vi "Disconnect.vi"(8 "Error In":errorcluster, 11 "Agent In":refnum<class "Agent.lvclass">) -> (0 "Error Out":errorcluster, 3 "Agent Out":refnum<class "Agent.lvclass">)   [LabVIEW 2018, in "Toolkit.lvlib" / "Agent.lvclass"]
doc: "Disconnects and closes the connection to the SSH agent application. This should be called before the Agent object is destroyed."
uses:
  Agent.lvclass
  Agent.lvclass/Agent.ctl
  Session/Session.lvclass/Session.ctl
  SSH/SSH.lvclass/SSH.ctl
  Toolkit.lvlib
  Session/Session.lvclass
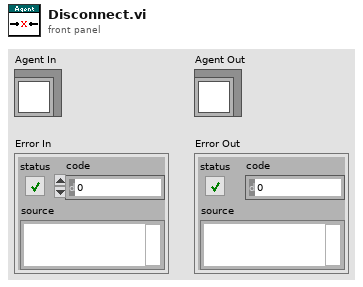
[diagram p1: front panel]
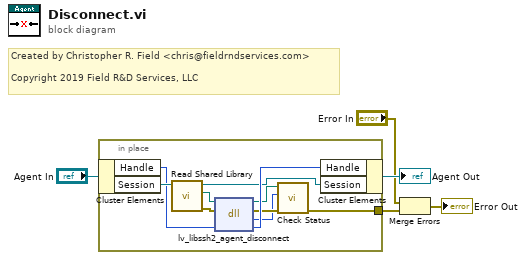
[diagram p0: block diagram]
diagram:
  # "Created by Christopher R. Field <chris@fieldrndservices.com>\n\nCopyright 2019 Field R&D Services, LLC"
  n1 = in-place {
    in-place-border: [w12] -> w5
    n2 = in-place-cluster #1("Agent In") -> ("Handle"=w7:u64, "Session"=w10:refnum<class "Session.lvclass">)
    n3 = call "Read Shared Library.vi"("Session In"=w10) -> ("Erorr Out"=w8:errorcluster, "libssh2lv Shared Library"=w9:path, "Session Out"=w6:refnum<class "Session.lvclass">)  [unwired: 8 in]
    n4 = dll-call lib="libssh2lv.*" fn="lv_libssh2_agent_disconnect"(path in=w9, error in=w8, "handle"=w7) -> (path out=w13:path, error out=w14:errorcluster, "result"=w11:i32, "handle"=w15:u64)  [unwired: 1 in]
    n5 = call "Check Status.vi"("Error In"=w14, "Status"=w11, "lv-libssh2 Shared Library In"=w13) -> ("Error Out"=w12:errorcluster)  [unwired: 7 in, 1 out]
    n6 = in-place-cluster #1("Handle"=w15, "Session"=w6) -> (→"Agent Out":refnum<class "Agent.lvclass">)
  }
  n7 = Merge Errors("Error In", w5) -> (→"Error Out":errorcluster)
